vi "test_decodeTxRxUDP config.vi"() -> ()   [LabVIEW 2020]
uses:
  <instrlib>/AIM GmbH/_AIM 664/_controls/comm_verification_rx.ctl
  <instrlib>/AIM GmbH/_AIM 664/_controls/comm_udp_rx.ctl
  <instrlib>/AIM GmbH/_AIM 664/_controls/comm_config_vl_tx.ctl
  <instrlib>/AIM GmbH/_AIM 664/_controls/comm_udp_tx.ctl
  Shared/Encoding (Arinc664).ctl
  <instrlib>/AIM GmbH/_AIM 664/AIM664LV.lvlib
panel:
  out "rx_param size":i32
  out "tx_udp_vl size":i32
  out "tx_param size":i32
  out "rx_udp_vl size":i32
  out "last mod 4":timestamp
  out "last mod 3":timestamp
  out "last mod 2":timestamp
  out "last mod":timestamp
  out "tx_param":T2(array[cluster]) {"Parameters"."encoding" items=["BNR", "BCD", "Discrete"]}
  out "rx_param":T2(array[cluster]) {"Parameters"."encoding" items=["BNR", "BCD", "Discrete"]}
  out "tx_udp_vl":T5(array[cluster]) {"VL Config"."NetSelect" items=["FDX_TX_FRAME_DLY_A"=0, "FDX_TX_FRAME_DLY_B"=1, "FDX_TX_FRAME_BOTH "=3, "FDX_TX_FRAME_ONLY_A"=4, "FDX_TX_FRAME_ONLY_B "=5]; "VL Config"."interfaceID" format="%.0b"}
  out "rx_udp_vl":T8(array[cluster]) {"VL Config"."FilterMode" items=["FDX_RX_VL_FLT_DIS", "FDX_RX_VL_FLT_ENA ", "FDX_RX_VL_FLT_ENA_INV"]; "VL Config"."VLBufSize" format="%.0x"; "VL Config"."VerificationMode" items=["FDX_RX_VL_CHECK_ENA_DEFAULT"=65535, "FDX_RX_VL_CHECK_REDMAM"=16, "DX_RX_VL_CHECK_TRAFIC"=8, "FDX_RX_VL_CHECK_FRAMESIZE"=4, "FDX_RX_VL_CHECK_SNINTEG"=2, "FDX_RX_VL_CHECK_INVPAC"=1, "FDX_RX_VL_CHECK_DISA"=0]}
  out "error out 4":errorcluster
  out "error out 3":errorcluster
  out "error out 2":errorcluster
  out "error out":errorcluster
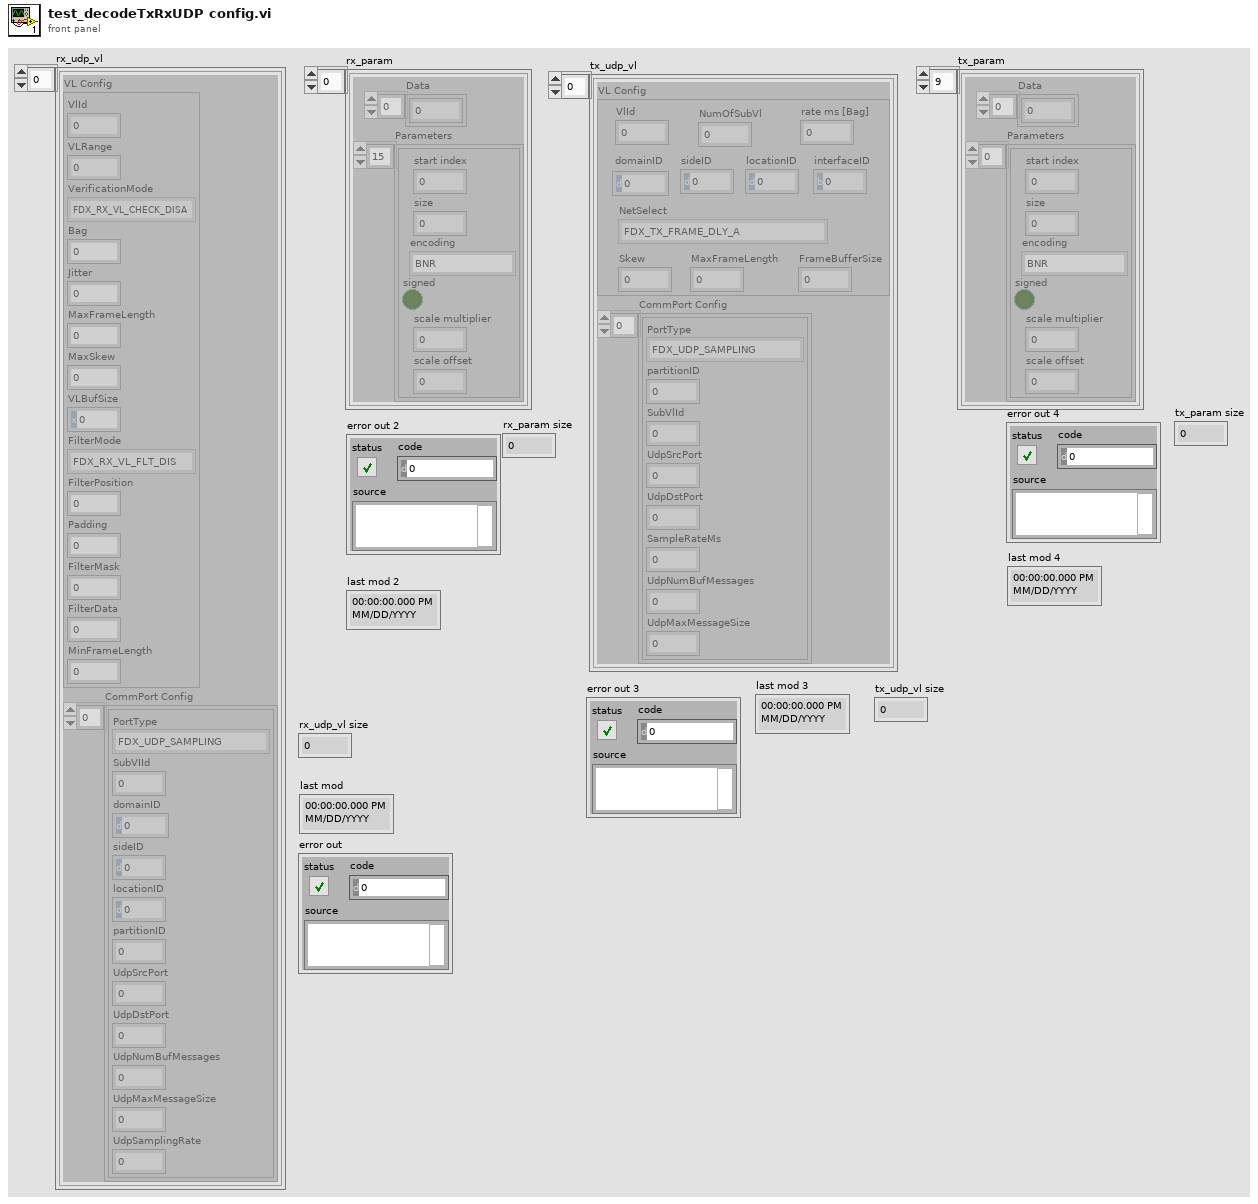
[diagram p1: front panel]
types:
  T1 = typedef "Encoding (Arinc664).ctl" = u16
  T2 = cluster{"Data":u8[], "Parameters":cluster{"start index":i32, "size":i32, "encoding":T1, "signed":bool, "scale multiplier":dbl, "scale offset":dbl}[]}[]
  T3 = typedef "AIM664LV.lvlib/comm_config_vl_tx.ctl" = cluster{"VlId":u16, "NumOfSubVl":u16, "rate ms [Bag]":u32, "domainID":u8, "sideID":u8, "locationID":u8, "interfaceID":u8, "NetSelect":u32, "Skew":u32, "MaxFrameLength":u32, "FrameBufferSize":u32}
  T4 = typedef "AIM664LV.lvlib/comm_udp_tx.ctl" = cluster{"PortType":enum16{"FDX_UDP_SAMPLING", "FDX_UDP_QUEUING"}, "partitionID":u8, "SubVlId":u8, "UdpSrcPort":u16, "UdpDstPort":u16, "SampleRateMs":dbl, "UdpNumBufMessages":u32, "UdpMaxMessageSize":u32}
  T5 = cluster{"VL Config":T3, "CommPort Config":T4[]}[]
  T6 = typedef "AIM664LV.lvlib/comm_verification_rx.ctl" = cluster{"VlId":u16, "VLRange":u32, "VerificationMode":u32, "Bag":u32, "Jitter":u32, "MaxFrameLength":u32, "MaxSkew":u32, "VLBufSize":u32, "FilterMode":u32, "FilterPosition":u32, "Padding":u32, "FilterMask":u32, "FilterData":u32, "MinFrameLength":u32}
  T7 = typedef "AIM664LV.lvlib/comm_udp_rx.ctl" = cluster{"PortType":enum16{"FDX_UDP_SAMPLING", "FDX_UDP_QUEUING"}, "SubVIId":u32, "domainID":u8, "sideID":u8, "locationID":u8, "partitionID":u8, "UdpSrcPort":u16, "UdpDstPort":u16, "UdpNumBufMessages":u32, "UdpMaxMessageSize":u32, "UdpSamplingRate":u32}
  T8 = cluster{"VL Config":T6, "CommPort Config":T7[]}[]
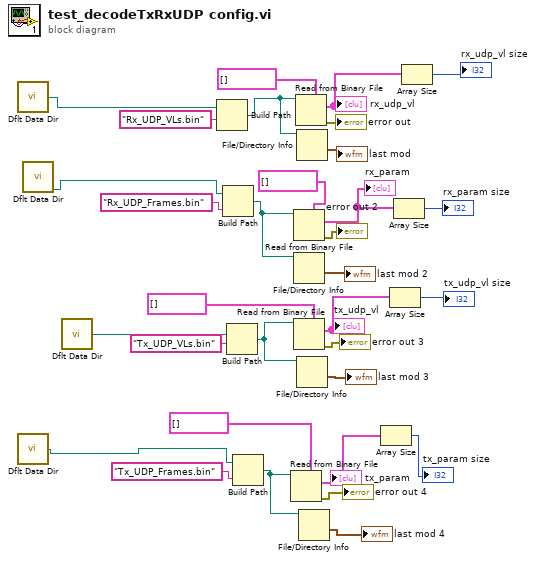
[diagram p0: block diagram]
diagram:
  n1 = call <vilib>:"Dflt Data Dir.vi"() -> ("App:Default Data Directory"=w28:path)
  n2 = call <vilib>:"Dflt Data Dir.vi"() -> ("App:Default Data Directory"=w18:path)
  n3 = call <vilib>:"Dflt Data Dir.vi"() -> ("App:Default Data Directory"=w20:path)
  n4 = call <vilib>:"Dflt Data Dir.vi"() -> ("App:Default Data Directory"=w19:path)
  n5 = Build Path(base path=w28, name or relative path="Rx_UDP_VLs.bin" ("format string")) -> (appended path=w16:path)
  n6 = Build Path(base path=w20, name or relative path="Rx_UDP_Frames.bin" ("format string")) -> (appended path=w11:path)
  n7 = Build Path(base path=w19, name or relative path="Tx_UDP_VLs.bin" ("format string")) -> (appended path=w10:path)
  n8 = Build Path(base path=w18, name or relative path="Tx_UDP_Frames.bin" ("format string")) -> (appended path=w17:path)
  n9 = Read from Binary File(5:T2 [] ("comm port payload"), 11:w17) -> (0:→"error out 4":errorcluster, 2:w1:T2)  [unwired: 4 in, 2 out]
  "tx_param" <- w1
  n10 = Read from Binary File(5:T2 [] ("CommPort Payload"), 11:w11) -> (0:→"error out 2":errorcluster, 2:w9:T2)  [unwired: 4 in, 2 out]
  "rx_param" <- w9
  n11 = File/Directory Info(path=w11) -> (last mod=→"last mod 2":timestamp)  [unwired: 1 in, 6 out]
  n12 = Read from Binary File(5:T5 [] ("VL configurations"), 11:w10) -> (0:→"error out 3":errorcluster, 2:w6:T5)  [unwired: 4 in, 2 out]
  "tx_udp_vl" <- w6
  n13 = Read from Binary File(5:T8 [] ("VL Configurations"), 11:w16) -> (0:→"error out":errorcluster, 2:w4:T8)  [unwired: 4 in, 2 out]
  "rx_udp_vl" <- w4
  n14 = File/Directory Info(path=w16) -> (last mod=→"last mod":timestamp)  [unwired: 1 in, 6 out]
  n15 = File/Directory Info(path=w10) -> (last mod=→"last mod 3":timestamp)  [unwired: 1 in, 6 out]
  n16 = File/Directory Info(path=w17) -> (last mod=→"last mod 4":timestamp)  [unwired: 1 in, 6 out]
  n17 = Array Size(array=w1) -> (size(s)=→"tx_param size":i32)
  n18 = Array Size(array=w6) -> (size(s)=→"tx_udp_vl size":i32)
  n19 = Array Size(array=w9) -> (size(s)=→"rx_param size":i32)
  n20 = Array Size(array=w4) -> (size(s)=→"rx_udp_vl size":i32)
